vi "RPI2 Main_ ADS1115.vi"() -> ()   [LabVIEW 2014]
uses:
  User Defined/I2C_Platform_Selector.ctl
  <vilib>/Platform/TimedLoop/XDataNode/timing_clust.ctl
  <vilib>/Platform/TimedLoop/XDataNode/nitl_modes.ctl
  <vilib>/Platform/TimedLoop/XDataNode/wakeup.ctl
  <vilib>/MakerHub/LINX/Public/Peripherals/Digital/Digital Write 1 Chan.vi
  <vilib>/MakerHub/LINX/Public/Peripherals/Digital/Digital Write N Chans.vi
  <vilib>/MakerHub/LINX/Private/Local IO/LinxDigitalWrite.vi
  <vilib>/MakerHub/LINX/Public/Utilities/Check Channel.vi
  <vilib>/MakerHub/LINX/Private/Local IO/Handle Errors.vi
  <vilib>/MakerHub/LINX/Public/Utilities/Open Local.vi
  <vilib>/MakerHub/LINX/Private/Utilties/Generate Error.vi
  <vilib>/platform/TimedLoop/XDataNode/XDataNode.xnode
  <vilib>/MakerHub/LINX/LMH-LINX.lvlib
  <vilib>/Platform/TimedLoop/XDataNode/XDNodeRunTimeDep.lvlib
panel:
  out "Scale Value (mV)":dbl
  out "Data":u8[](array[numeric]) format="%.0x"
  out "(hi.lo)":u16 format="%.0x"
  out "uA out":dbl
  in  "Stop Button":bool
  in  "DO Channel":u8
  in  "Output Value 2":bool
  in  "DO Channel 2":u8
  in  "Output Value":bool
  in  "Level":bool
  in  "Stop Button 3":bool
  out "Waveform Chart":dbl(graph)
  # "CH1 - uA\nCH2 - mA\nCH3 - VCC 2.8/2"
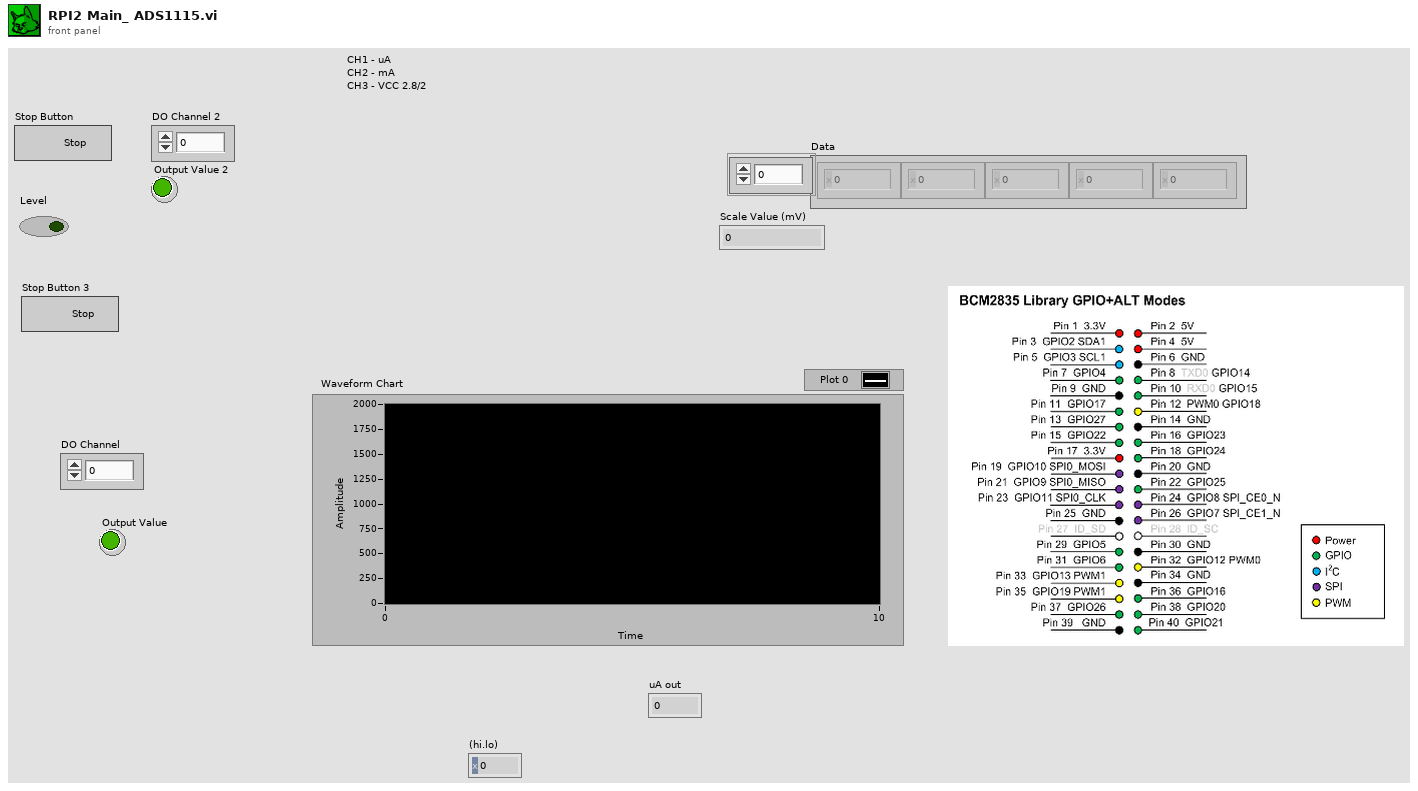
[diagram p1: front panel]
types:
  T1 = typedef "I2C_Platform_Selector.ctl" = enum16{"ESP8266-I2C", "Raspberry Pi-I2C"}
  T2 = cluster{"ADS1015-Channel Selector":enum8{"DIFF-AI0-AI1", "DIFF-AI0-AI3", "DIFF-AI1-AI3", "DIFF-AI2-AI3", "Single Ended - AI0", "Single Ended - AI1", "Single Ended - AI2", "Single Ended - AI3"}, "ADS1015 -Gain & Scale":enum8{"FS=+/-6.144 V", "FS=+/-4.096 V", "FS=+/-2.048 V", "FS=+/-1.024 V", "FS=+/-0.512 V", "FS=+/-0.256-A V", "FS=+/-0.256-B V", "FS=+/-0.256-C V"}, "ADS1015- Acquire Mode":enum16{"Continuous Conversion Mode", "Single Shot Mode"}, "ADS1015 Sample Rate":enum8{"128 SPS", "250 SPS", "490 SPS", "920 SPS", "1600 SPS", "2400 SPS", "3300 SPS", "3300 SPS A"}}
  T3 = typedef "LMH-LINX.lvlib/LINX Ref.ctl" = cluster{"IO":T4, "Interface":T5, "LINX Device Config":T6}
  T4 = typedef "LMH-LINX.lvlib/Platform.ctl" = enum16{"Remote", "Local"}
  T5 = typedef "LMH-LINX.lvlib/Interface.ctl" = enum16{"Serial", "TCP"}
  T6 = typedef "LMH-LINX.lvlib/Device.lvlib/LINX Device Config.ctl" = cluster{"Interface":T5, "COM Port":refnum<visa-resource-name>, "TCP Configuration":T7, "Device Family":u8, "Device ID":u8, "Device Name":string, "TCP Ref":refnum<k5>, "Channels":T8}
  T7 = typedef "LMH-LINX.lvlib/Device.lvlib/TCP Config.ctl" = cluster{"IP Address":string, "Port":u16}
  T8 = typedef "LMH-LINX.lvlib/Channels.ctl" = cluster{"DI":u8[], "DO":u8[], "AI":u8[], "AO":u8[], "PWM":u8[], "QE":u8[], "UART":u8[], "I2C 2":u8[], "SPI":u8[], "CAN":u8[], "Servo":u8[], "AI Ref (V)":dbl, "AI Resolution (Bits)":u8, "AO Ref (V)":dbl, "AO Resolution (Bits)":u8}
  T9 = enum8{"FS=+/-6.144 V", "FS=+/-4.096 V", "FS=+/-2.048 V", "FS=+/-1.024 V", "FS=+/-0.512 V", "FS=+/-0.256-A V", "FS=+/-0.256-B V", "FS=+/-0.256-C V"}
  T10 = typedef "XDNodeRunTimeDep.lvlib/timing_clust.ctl" = cluster{"Expected End [f-1]":u64, "Actual End [f-1]":u64, "Finished Late? [f-1]":bool, "Expected End [i-1]":u64, "Actual End [i-1]":u64, "Finished Late? [i-1]":bool, "Expected Start [i]":u64, "Actual Start [i]":u64, "Expected Start [f]":u64, "Actual Start [f]":u64, "Source Name":string, "Structure Name":string, "Period":i64, "Deadline":i64, "Offset":i64, "Start":i64, "Priority":i32, "Timeout":i32, "Mode":T11, "Wakeup Reason":T12, "Error":errorcluster, "Source Type":string, "Secondary Source Type":string, "Global End Time":u64, "Global Start Time":u64, "Frame Duration":u64, "Iteration Duration":u64, "Assigned CPU":i32, "I/O Scan Engine Mode":u32}
  T11 = typedef "XDNodeRunTimeDep.lvlib/nitl_modes.ctl" = enum32{"No Change", "Process missed periods, maintain original phase", "Discard missed periods, maintain original phase", "Process missed periods, ignore original phase", "Discard missed periods, ignore original phase"}
  T12 = typedef "XDNodeRunTimeDep.lvlib/wakeup.ctl" = enum32{"Normal", "Aborted", "Asynchronous wakeup", "Timing source error", "Timed loop error", "Timeout"}
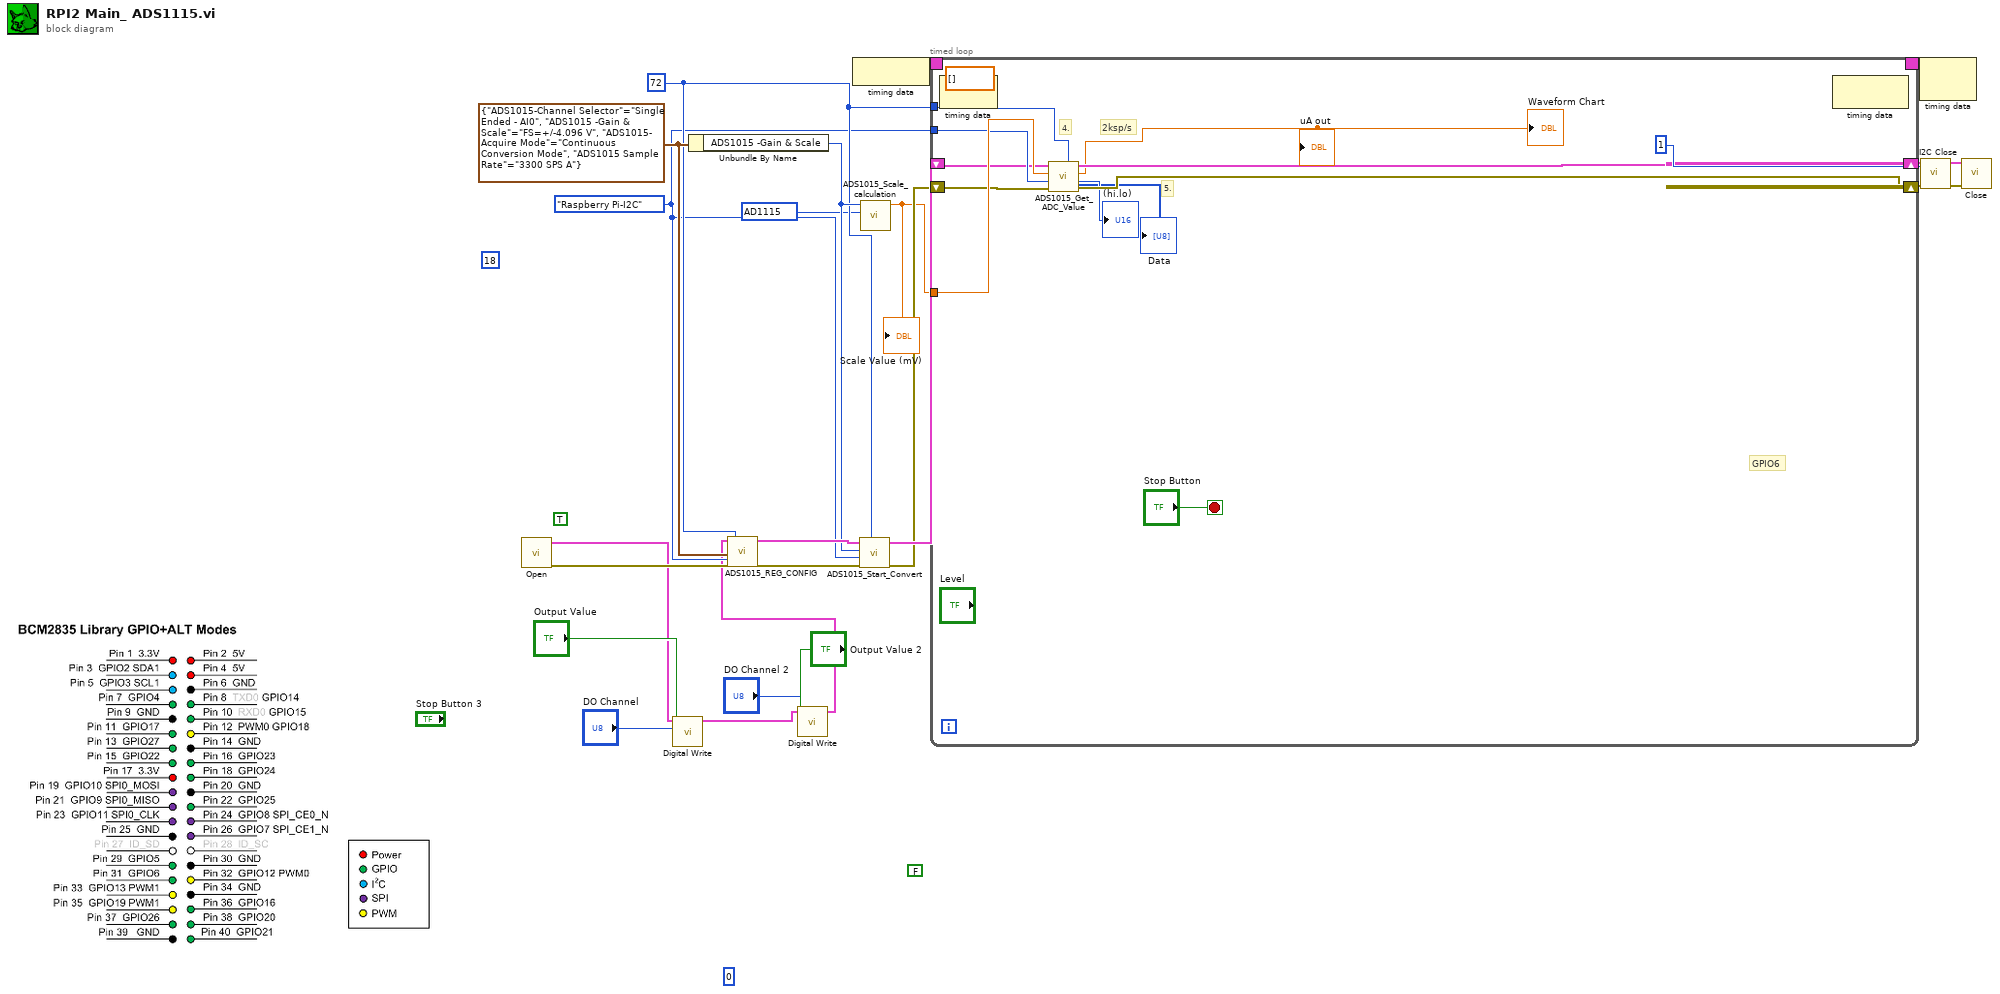
[diagram p0: block diagram]
diagram:
  w1 = 65536 items=["ADS1015"=4096, "AD1115"=65536] ("IC Selector")
  (unwired) FALSE
  (unwired) 0 ("bytes written")
  (unwired) u8 18 ("DI Channel 2")
  (unwired) TRUE ("Output Value")
  w14 = I2C_Platform_Selector."Raspberry Pi-I2C" ("I2C_Channel_platform")
  w15 = u8 72 ("I2C Slave Address (0)")
  w22 = T2 {"ADS1015-Channel Selector"=enum."Single Ended - AI0", "ADS1015 -Gain & Scale"=enum."FS=+/-4.096 V", "ADS1015- Acquire Mode"=enum."Continuous Conversion Mode", "ADS1015 Sample Rate"=enum."3300 SPS A"} ("ADS1015 Reg Config")
  n1 = call-poly <vilib>:"Open.vi"() -> ("Error Out"=w10:errorcluster, "LINX Resource"=w4:T3)  [unwired: 9 in, 1 out]
  n2 = call-poly <vilib>:"Digital Write.vi"("Output Value"="Output Value", "DO Channel"="DO Channel", "LINX Resource"=w4) -> ("LINX Resource"=w5:T3)  [unwired: 7 in, 1 out]
  n3 = Unbundle By Name(w22) -> ("ADS1015 -Gain & Scale"=w21:T9)
  n4 = call-poly <vilib>:"Digital Write.vi"("Output Value"="Output Value 2", "DO Channel"="DO Channel 2", "LINX Resource"=w5) -> ("LINX Resource"=w3:T3)  [unwired: 7 in, 1 out]
  n5 = call "ADS1015_REG_CONFIG.vi"("LINX Resource in"=w3, "ADS1015 Reg Config"=w22, "I2C_Channel_platform"=w14, "Error In"=w10, "I2C Slave Address (0)"=w15) -> ("LINX Resource out"=w24:T3, "Error Out"=w25:errorcluster)  [unwired: 13 in]
  n6 = node-c288() -> (w13:T10)
  n7 = call "ADS1015_Start_Convert.vi"("I2C Slave Address (0)"=w15, "error in (no error)"=w25, "I2C_Channel_platform"=w14, "Scale mV"=w21, "LINX Resource in"=w24) -> ("error out"=w11:errorcluster, "LINX Resource out"=w23:T3)  [unwired: 4 in, 1 out]
  n8 = call "ADS1015_Scale_calculation.vi"("IC Selector"=w1, "ADS1015 -Gain & Scale"=w21) -> ("Scale Value (mV)"=w2:dbl)  [unwired: 9 in]
  "Scale Value (mV)" <- w2
  n9 = timed-loop {
    tunnel: w2 -> [w36]
    tunnel: w15 -> [w34]
    tunnel: w14 -> [w33]
    shift-right: [w31] -> w17
    shift-left: w11 -> [w32]
    shift-right: [w35] -> w19
    shift-left: w23 -> [w28]
    timing: w13 -> [_]
    timing-out: [_] -> w12
    stop <- "Stop Button" stop-if-true
    (unwired) dbl[] []
    # "GPIO6"
    # "2ksp/s"
    # "5."
    # "4."
    n10 = node-c288() -> ()  [unwired: 1 in, 1 out]
    n11 = call "ADS1015_Get_ADC_Value.vi"("I2C Slave Address (0)"=w34, "error in (no error)"=w32, "I2C_Channel_platform"=w33, "Scale Value (mV)"=w36, "LINX Resource in"=w28) -> ("error out"=w31:errorcluster, "(hi.lo)"=→"(hi.lo)":u16, "mV out"=→"Waveform Chart" →"uA out":dbl, "LINX Resource"=w35:T3, "Data"=→"Data":u8[])  [unwired: 2 in]
    n12 = node-c288() -> ()  [unwired: 1 in, 1 out]
  }
  n13 = node-c288(w12) -> ()  [unwired: 1 out]
  n14 = call <vilib>:"I2C Close.vi"("I2C Channel (0)"=u8 1, "Error In"=w17, "LINX Resource"=w19) -> ("Error Out"=w16:errorcluster, "LINX Resource"=w18:T3)  [unwired: 7 in]
  n15 = call <vilib>:"Close.vi"("Error In"=w16, "LINX Resource"=w18) -> ()  [unwired: 9 in, 1 out]
